vi "Siargo Initialization.vi"(8 "error in (no error)":errorcluster, 11 "VISA resource name":refnum<visa-resource-name>) -> (0 "error out":errorcluster, 3 "serial master instance":refnum<class "Modbus Master.lvclass">)   [LabVIEW 2020]
uses:
  <vilib>/NI/Modbus Library/API/Master/Modbus Master.lvclass
  <vilib>/NI/Modbus Library/API/Wrapper/Create Serial Master.vi
  <vilib>/NI/Modbus Library/API/Wrapper/API Main.lvlib
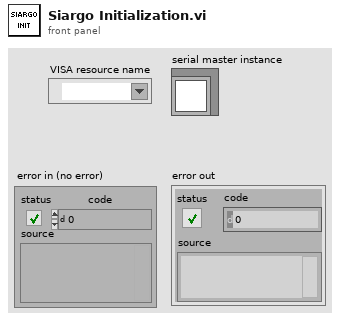
[diagram p1: front panel]
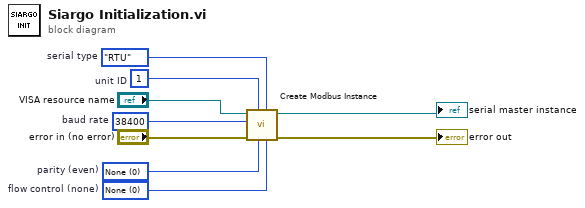
[diagram p0: block diagram]
diagram:
  w9 = u16 0 items=["None", "XON/XOFF", "RTS/CTS", "XON/XOFF & RTS/CTS", "DTR/DSR", "XON/XOFF & DTR/DSR"]  # flow control (none)
  w8 = u16 0 items=["None", "Odd", "Even", "Mark", "Space"]  # parity (even)
  w3 = u8 1  # unit ID
  w7 = enum16{"RTU", "ASCII"}."RTU"  # serial type
  w6 = u32 38400  # baud rate
  n1 = call-poly <vilib>:"Create Modbus Instance.vi"("flow control (none)"=w9, "serial type"=w7, "parity (even)"=w8, "unit ID"=w3, "error in"="error in (no error)", "baud rate"=w6, "VISA resource name"="VISA resource name") -> ("error out"=→"error out":errorcluster, "serial master instance"=→"serial master instance":refnum<class "Modbus Master.lvclass">)  [unwired: 3 in]
